vi "Is target close to current.vi"(9 "Current Position":dbl, 10 "Target Position":dbl, 11 "Acceptable Error":dbl) -> (3 "Acceptable":bool)   [LabVIEW 2019]
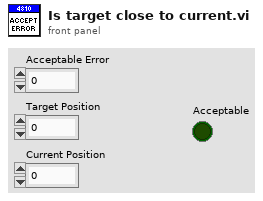
[diagram p1: front panel]
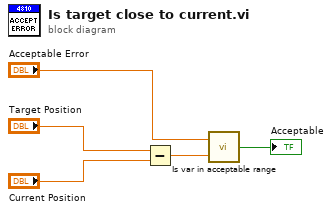
[diagram p0: block diagram]
diagram:
  n1 = Subtract(x="Target Position", y="Current Position") -> (x-y=w3:dbl)
  n2 = call "Is var in acceptable range.vi"("Variable"=w3, "Acceptable plus minus"="Acceptable Error") -> ("Acceptable"=→"Acceptable":bool)
